vi "Proceed.vi"(7 "component is ready (Y)":bool=TRUE, 8 "error in (no error)":errorcluster, 10 "ProceedMessage":refnum<class "ProceedMessage.lvclass">, 11 "DAQOrcaFlash in":refnum<class "DAQOrcaFlash.lvclass">) -> (0 "error out":errorcluster, 2 "all observers are ready?":bool, 3 "DAQOrcaFlash out":refnum<class "DAQOrcaFlash.lvclass">)   [LabVIEW 2012, in "DAQOrcaFlash.lvclass"]
uses:
  DAQOrcaFlash.lvclass
  <vilib>/Distrio/Murmex/ProceedMessage/ProceedMessage.lvclass
  DAQOrcaFlash.lvclass/DAQOrcaFlash.ctl
  <vilib>/Distrio/Murmex/Murmex/Murmex.lvclass
panel:
  # "This method is called when the PROCEED\ntrigger is sent. \n\nOverride this method when your component needs to\nrespond to this trigger. \n\nCall parent for proper implementation"
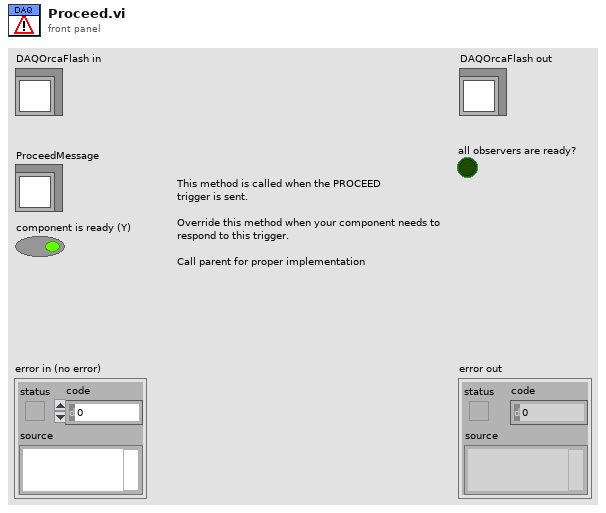
[diagram p1: front panel]
types:
  T1 = typedef "DAQOrcaFlash.lvclass/imaging_mode.ctl" = enum16{"focus mode", "single sweep"}
  T2 = typedef "IMAQ Image.ctl" = refnum<image>
  T3 = cluster{"width":u32, "height":u32, "datatype":u32}
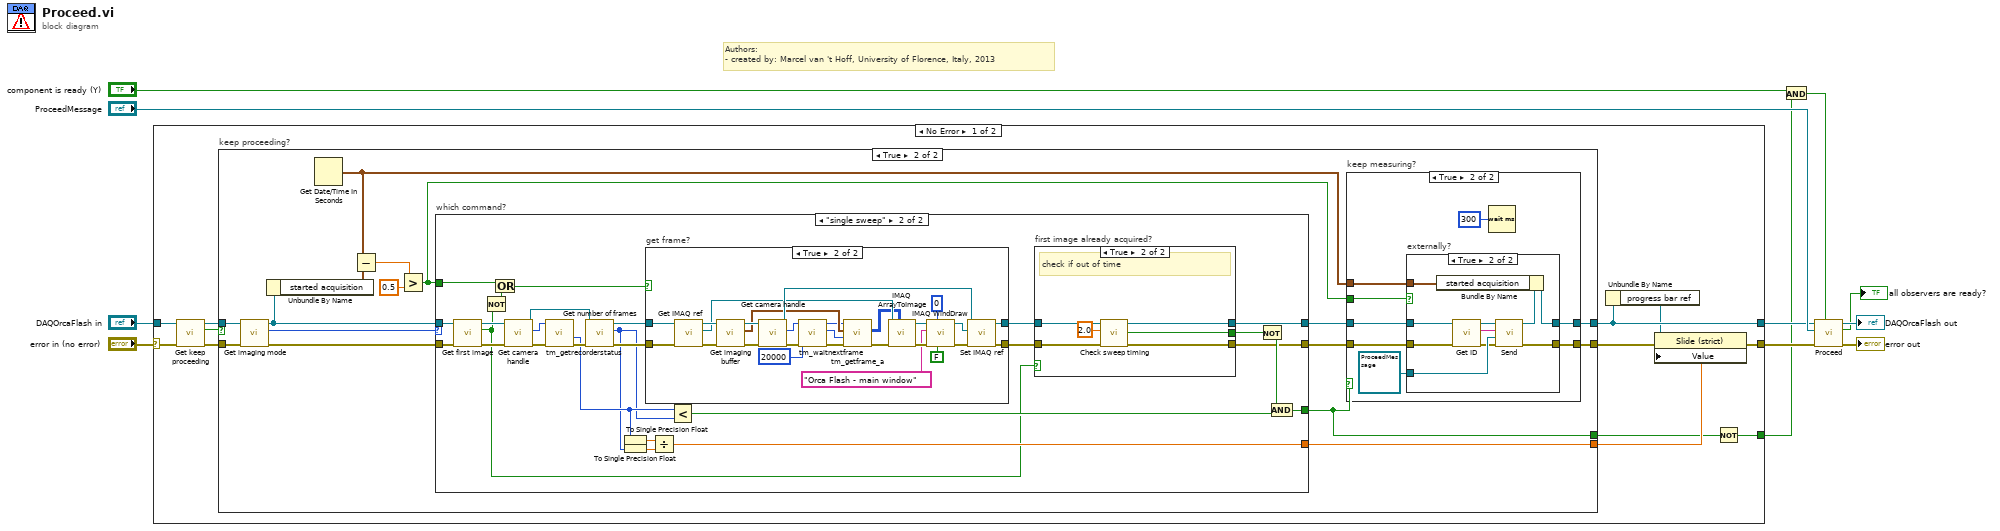
[diagram p0: block diagram]
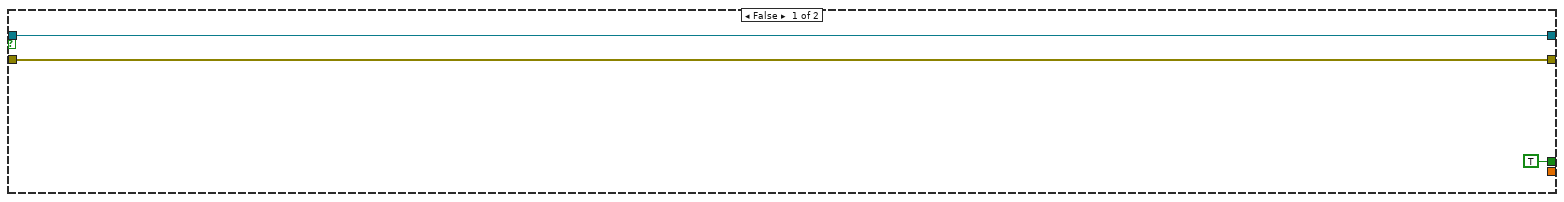
[diagram p2: hidden frame]
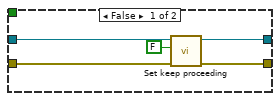
[diagram p3: hidden frame]
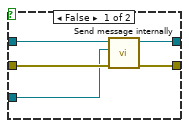
[diagram p4: hidden frame]
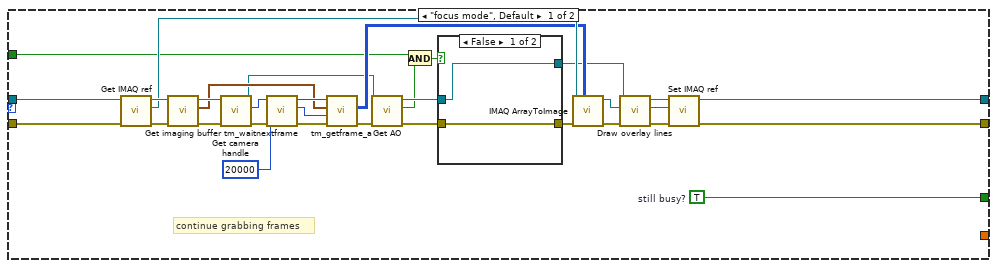
[diagram p5: hidden frame]
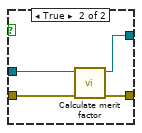
[diagram p6: hidden frame]
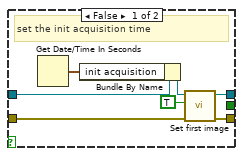
[diagram p7: hidden frame]
diagram:
  # "Authors: \n- created by: Marcel van 't Hoff, University of Florence, Italy, 2013"
  n1 = case shown="No Error" "error in (no error)" {
    selector: "error in (no error)" -> [w15 w178]
    tunnel: [w20 w178] -> w6
    tunnel: [w23 w177] -> w5
    tunnel: "DAQOrcaFlash in" -> [w16 w177]
    tunnel: [w17 _] -> w3
    frame No Error {
      n2 = call-dynamic "Get keep proceeding.vi"("error in (no error)"=w15, "DAQOrcaFlash in"=w16) -> ("error out"=w14:errorcluster, "keep proceeding?"=w12:bool, "DAQOrcaFlash out"=w13:refnum<class "DAQOrcaFlash.lvclass">)  [unwired: 7 in]
      n3 = case "keep proceeding?" shown="True" w12 {
        tunnel: [w25 w36] -> w19
        tunnel: [w26 w37] -> w23
        tunnel: w13 -> [w26 w40]
        tunnel: w14 -> [w25 w39]
        tunnel: [_ w38] -> w21
        tunnel: [TRUE ("proceed?") w29] -> w18
        frame False {
        }
        frame True {
          n4 = call "Get imaging mode.vi"("error in (no error)"=w39, "DAQMH121119OrcaFlash in"=w40) -> ("error out"=w42:errorcluster, "imaging mode"=w41:T1, "DAQMH121119OrcaFlash out"=w32:refnum<class "DAQOrcaFlash.lvclass">)  [unwired: 7 in]
          n5 = Unbundle By Name(w32) -> ("started acquisition"=w33:timestamp)
          n6 = Get Date/Time In Seconds() -> (seconds since 1Jan1904=w31:timestamp)
          n7 = Subtract(x=w31, y=w33) -> (x-y=w34:dbl)
          n8 = Greater?(x=w34, y=0.5) -> (0:w30:bool)
          n9 = case "which command?" shown="\"single sweep\"" w41 {
            tunnel: w42 -> [w101 w135]
            tunnel: w32 -> [w102 w119]
            tunnel: [w100 w113] -> w27
            tunnel: [w99 w112] -> w28
            tunnel: [_ w126] -> w38
            tunnel: [w98 w121] -> w29
            tunnel: w30 -> [w79 w117]
            frame "focus mode", Default {
              w98 = TRUE  # still busy?
              # "continue grabbing frames"
              n10 = call "Get IMAQ ref.vi"("error in (no error)"=w101, "DAQMH121119OrcaFlash in"=w102) -> ("error out"=w93:errorcluster, "IMAQ reference"=w87:T2, "DAQMH121119OrcaFlash out"=w95:refnum<class "DAQOrcaFlash.lvclass">)  [unwired: 7 in]
              n11 = call "Get imaging buffer.vi"("error in (no error)"=w93, "DAQMH121119OrcaFlash in"=w95) -> ("error out"=w92:errorcluster, "imaging buffer"=w89:T3, "DAQMH121119OrcaFlash out"=w94:refnum<class "DAQOrcaFlash.lvclass">)  [unwired: 5 in, 2 out]
              n12 = call "Get camera handle.vi"("error in (no error)"=w92, "DAQMH121119OrcaFlash in"=w94) -> ("error out"=w96:errorcluster, "cam handle"=w97:u32, "DAQMH121119OrcaFlash out"=w82:refnum<class "DAQOrcaFlash.lvclass">)  [unwired: 7 in]
              n13 = call <userlib>:"tm_waitnextframe.vi"("error in (no error)"=w96, "Timeout"=20000, "Handle in"=w97) -> ("error out"=w91:errorcluster, "Frame Index"=w88:i32, "Handle out"=w90:u32)  [unwired: 5 in, 1 out]
              n14 = call <userlib>:"tm_getframe_a.vi"("error in (no error)"=w91, "Frame Index"=w88, "Buffer Info"=w89, "Handle in"=w90) -> ("error out"=w84:errorcluster, "Data 16"=w85:u16[][])  [unwired: 3 in, 3 out]
              n15 = call-dynamic "Get AO.vi"("error in (no error)"=w84, "DAQOrcaFlash in"=w82) -> ("error out"=w83:errorcluster, "AO"=w80:bool, "DAQOrcaFlash out"=w81:refnum<class "DAQOrcaFlash.lvclass">)  [unwired: 7 in]
              n16 = And(x=w79, y=w80) -> (x .and. y?=w78:bool)
              n17 = case shown="False" w78 {
                tunnel: [w104 w108] -> w86
                tunnel: w83 -> [w104 w105]
                tunnel: w81 -> [w103 w106]
                tunnel: [w103 w107] -> w72
                frame False {
                }
                frame True {
                  n18 = call-dynamic "Calculate merit factor.vi"("error in (no error)"=w105, "DAQOrcaFlash in"=w106) -> ("error out"=w108:errorcluster, "DAQOrcaFlash out"=w107:refnum<class "DAQOrcaFlash.lvclass">)  [unwired: 8 in]
                }
              }
              n19 = call "IMAQ ArrayToImage"("Image Pixels (U16)"=w85, "error in (no error)"=w86, "Image"=w87) -> ("error out"=w77:errorcluster, "Image Out"=w75:T2)  [unwired: 7 in]
              n20 = call "Draw overlay lines.vi"("error in (no error)"=w77, "IMAQ reference"=w75, "DAQOrcaFlash in"=w72) -> ("error out"=w76:errorcluster, "IMAQ reference out"=w74:T2, "DAQOrcaFlash out"=w73:refnum<class "DAQOrcaFlash.lvclass">)  [unwired: 6 in]
              n21 = call "Set IMAQ ref.vi"("error in (no error)"=w76, "IMAQ reference"=w74, "DAQMH121119OrcaFlash in"=w73) -> ("error out"=w100:errorcluster, "DAQMH121119OrcaFlash out"=w99:refnum<class "DAQOrcaFlash.lvclass">)  [unwired: 7 in]
            }
            frame "single sweep" {
              n22 = call-dynamic "Get first image.vi"("error in (no error)"=w135, "DAQOrcaFlash in"=w119) -> ("error out"=w120:errorcluster, "first image acquired?"=w115:bool, "DAQOrcaFlash out"=w118:refnum<class "DAQOrcaFlash.lvclass">)  [unwired: 7 in]
              n23 = Not(x=w115) -> (.not. x?=w109:bool)
              n24 = Or(x=w117, y=w109) -> (x .or. y?=w116:bool)
              n25 = call "Get camera handle.vi"("error in (no error)"=w120, "DAQMH121119OrcaFlash in"=w118) -> ("error out"=w134:errorcluster, "cam handle"=w133:u32, "DAQMH121119OrcaFlash out"=w132:refnum<class "DAQOrcaFlash.lvclass">)  [unwired: 7 in]
              n26 = call <userlib>:"tm_getrecorderstatus.vi"("error in (no error)"=w134, "Handle"=w133) -> ("error out"=w131:errorcluster, "Count"=w125:i32)  [unwired: 6 in, 2 out]
              n27 = call "Get number of frames.vi"("error in (no error)"=w131, "DAQMH121119OrcaFlash in"=w132) -> ("error out"=w130:errorcluster, "no. of frames"=w124:i32, "DAQMH121119OrcaFlash out"=w129:refnum<class "DAQOrcaFlash.lvclass">)  [unwired: 7 in]
              n28 = To Single Precision Float(number=w125) -> (single precision float=w127:sgl)
              n29 = To Single Precision Float(number=w124) -> (single precision float=w128:sgl)
              n30 = case "get frame?" shown="True" w116 {
                tunnel: w130 -> [w150 w168]
                tunnel: w129 -> [w149 w167]
                tunnel: [w149 w165] -> w110
                tunnel: [w150 w166] -> w114
                frame False {
                }
                frame True {
                  n31 = call "Get IMAQ ref.vi"("error in (no error)"=w168, "DAQMH121119OrcaFlash in"=w167) -> ("error out"=w175:errorcluster, "IMAQ reference"=w170:T2, "DAQMH121119OrcaFlash out"=w172:refnum<class "DAQOrcaFlash.lvclass">)  [unwired: 7 in]
                  n32 = call "Get imaging buffer.vi"("error in (no error)"=w175, "DAQMH121119OrcaFlash in"=w172) -> ("error out"=w176:errorcluster, "imaging buffer"=w164:T3, "DAQMH121119OrcaFlash out"=w174:refnum<class "DAQOrcaFlash.lvclass">)  [unwired: 5 in, 2 out]
                  n33 = call "Get camera handle.vi"("error in (no error)"=w176, "DAQMH121119OrcaFlash in"=w174) -> ("error out"=w160:errorcluster, "cam handle"=w163:u32, "DAQMH121119OrcaFlash out"=w173:refnum<class "DAQOrcaFlash.lvclass">)  [unwired: 7 in]
                  n34 = call <userlib>:"tm_waitnextframe.vi"("error in (no error)"=w160, "Timeout"=20000, "Handle in"=w163) -> ("error out"=w159:errorcluster, "Frame Index"=w161:i32, "Handle out"=w162:u32)  [unwired: 5 in, 1 out]
                  n35 = call <userlib>:"tm_getframe_a.vi"("error in (no error)"=w159, "Frame Index"=w161, "Buffer Info"=w164, "Handle in"=w162) -> ("error out"=w171:errorcluster, "Data 16"=w169:u16[][])  [unwired: 3 in, 3 out]
                  n36 = call "IMAQ ArrayToImage"("Image Pixels (U16)"=w169, "error in (no error)"=w171, "Image"=w170) -> ("error out"=w158:errorcluster, "Image Out"=w156:T2)  [unwired: 7 in]
                  n37 = call "IMAQ WindDraw"("Resize to Image Size? (Y)"=FALSE, "Window Number (0...15)"=0, "error in (no error)"=w158, "Title"="Orca Flash - main window", "Image"=w156) -> ("error out"=w157:errorcluster, "Image Out (duplicate)"=w155:T2)  [unwired: 5 in]
                  n38 = call "Set IMAQ ref.vi"("error in (no error)"=w157, "IMAQ reference"=w155, "DAQMH121119OrcaFlash in"=w173) -> ("error out"=w166:errorcluster, "DAQMH121119OrcaFlash out"=w165:refnum<class "DAQOrcaFlash.lvclass">)  [unwired: 7 in]
                }
              }
              n39 = Divide(x=w127, y=w128) -> (x/y=w126:sgl)
              n40 = Less?(x=w125, y=w124) -> (x < y?=w122:bool)
              n41 = case "first image already acquired?" shown="True" w115 {
                tunnel: w114 -> [w138 w147]
                tunnel: [w137 w146] -> w113
                tunnel: [w139 w145] -> w112
                tunnel: [_ w144] -> w111
                tunnel: w110 -> [w142 w143]
                frame False {
                  # "set the init acquisition time"
                  n42 = Get Date/Time In Seconds() -> (seconds since 1Jan1904=w141:timestamp)
                  n43 = Bundle By Name(cluster=w142, "init acquisition"=w141) -> (w140:refnum<class "DAQOrcaFlash.lvclass">)
                  n44 = call-dynamic "Set first image.vi"("error in (no error)"=w138, "first image acquired?"=TRUE, "DAQOrcaFlash in"=w140) -> ("error out"=w137:errorcluster, "DAQOrcaFlash out"=w139:refnum<class "DAQOrcaFlash.lvclass">)  [unwired: 7 in]
                }
                frame True {
                  # "check if out of time"
                  n45 = call-dynamic "Check sweep timing.vi"("error in (no error)"=w147, "Tolerance (s)"=2.0, "DAQOrcaFlash in"=w143) -> ("error out"=w146:errorcluster, "out of time?"=w144:bool, "DAQOrcaFlash out"=w145:refnum<class "DAQOrcaFlash.lvclass">)  [unwired: 6 in]
                }
              }
              n46 = Not(x=w111) -> (.not. x?=w123:bool)
              n47 = And(x=w123, y=w122) -> (x .and. y?=w121:bool)
            }
          }
          n48 = case "keep measuring?" shown="True" w29 {
            tunnel: w27 -> [w47 w50]
            tunnel: [w46 w53] -> w36
            tunnel: w28 -> [w45 w55]
            tunnel: [w44 w54] -> w37
            tunnel: w30 -> [_ w52]
            tunnel: w31 -> [_ w51]
            frame False {
              n49 = call-dynamic "Set keep proceeding.vi"("error in (no error)"=w47, "keep proceeding?"=FALSE, "DAQOrcaFlash in"=w45) -> ("error out"=w46:errorcluster, "DAQOrcaFlash out"=w44:refnum<class "DAQOrcaFlash.lvclass">)  [unwired: 7 in]
            }
            frame True {
              n50 = case "externally?" shown="True" w52 {
                tunnel: w50 -> [w60 w66]
                tunnel: refnum<class "ProceedMessage.lvclass"> refnum ("ProceedMessage") -> [w59 w68]
                tunnel: w55 -> [w58 w69]
                tunnel: [w57 w61] -> w54
                tunnel: [w56 w70] -> w53
                tunnel: w51 -> [_ w63]
                frame False {
                  n51 = call <vilib>:"Send message internally.vi"("error in (no error)"=w60, "Message"=w59, "Murmex in"=w58) -> ("error out"=w56:errorcluster, "Murmex out"=w57:refnum<class "DAQOrcaFlash.lvclass">)  [unwired: 7 in]
                }
                frame True {
                  n52 = call <vilib>:"Get ID.vi"("error in (no error)"=w66, "Murmex in"=w69) -> ("error out"=w65:errorcluster, "component id"=w64:string, "Murmex out"=w67:refnum<class "DAQOrcaFlash.lvclass">)  [unwired: 7 in]
                  n53 = call <vilib>:"Send.vi"("error in (no error)"=w65, "Message"=w68, "recipient"=w64, "Murmex in"=w67) -> ("error out"=w70:errorcluster, "Murmex out"=w62:refnum<class "DAQOrcaFlash.lvclass">)  [unwired: 6 in]
                  n54 = Bundle By Name(cluster=w62, "started acquisition"=w63) -> (w61:refnum<class "DAQOrcaFlash.lvclass">)
                }
              }
              n55 = Wait (ms)(milliseconds to wait=u32 300) -> ()  [unwired: 1 out]
            }
          }
        }
      }
      n56 = Unbundle By Name(w23) -> ("progress bar ref"=w22:refnum<vi>)
      n57 = property class="Slide (strict)"(reference=w22, error in=w19, "Value"=w21) -> (error out=w20:errorcluster)  [unwired: 1 out]
      n58 = Not(x=w18) -> (.not. x?=w17:bool)
    }
    frame Error {
    }
  }
  n59 = And(x="component is ready (Y)", y=w3) -> (x .and. y?=w2:bool)
  n60 = call-parent "Proceed.vi"("component is ready (Y)"=w2, "error in (no error)"=w6, "ProceedMessage"="ProceedMessage", "Murmex in"=w5) -> ("error out"=→"error out":errorcluster, "all observers are ready?"=→"all observers are ready?":bool, "Murmex out"=→"DAQOrcaFlash out":refnum<class "DAQOrcaFlash.lvclass">)  [unwired: 5 in]
